vi "XNode Template Single.vi"(0 "failure in":T1 {"code" format="%.0x"}, 1 "Tag":string, 5 "Data Type":variant) -> (4 "failure out":T1 {"code" format="%.0x"}, 6 "Value":dbl, 8 "failed":bool)   [LabVIEW 2013, in "Read Exception Property.xnode"]
doc: "This VI is used to read data stored in a Variant Repository, similar to a look up table. This VI is will get an attribute of the <b>Variant Repository In</b>, with the tag name of <b>Tag</b>, and return its value on <b>Value</b>, and then return the same varient data on <b>Varient Repository Out</b>. This VI will put an error on the <b>error out</b> if the tag is not found, there is no tag when needed, or the tag was found, but of the wrong data type.\n\nRight click and Select Type for simple data types, or choose Automatic and wire in the <b>Data Type</b> to be read. If Automatic is selected, and nothing is wired to the Data Type, the type can come from the sink of the wire wired to the Value terminal.\n\nIf the a Data Type terminal is not wired, then the <b>Tag</b> must also be provided. If the data type is selected using the <b>Data Type</b> input then the tag is optional, and if empty the label associated with the data passed in will be used as the tag.\n\nReading multiple tags can be done by right clicking and choosing Read Multiple Tags.\n\n-------------\nBrian Hoover (Hooovahh)\n\nProduct Name: Variant Repository\nPackage File Name: lava_lib_variant_repository\nPackage Version: 1.0.1.11\nMinimum LabVIEW Version: 11.0"
uses:
  Read Exception Property.xnode
  failure.ctl
  <vilib>/Utility/VariantDataType/VariantType.lvlib
  failure.lvlib
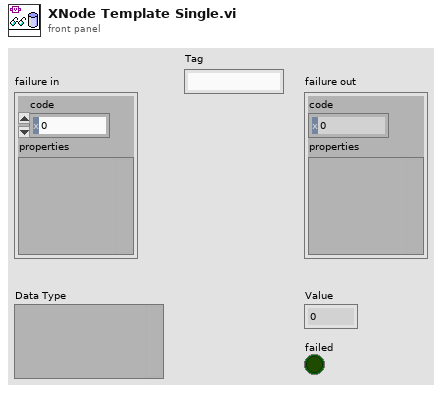
[diagram p1: front panel]
types:
  T1 = typedef "failure.lvlib/failure.ctl" = cluster{"code":i32, "properties":variant}
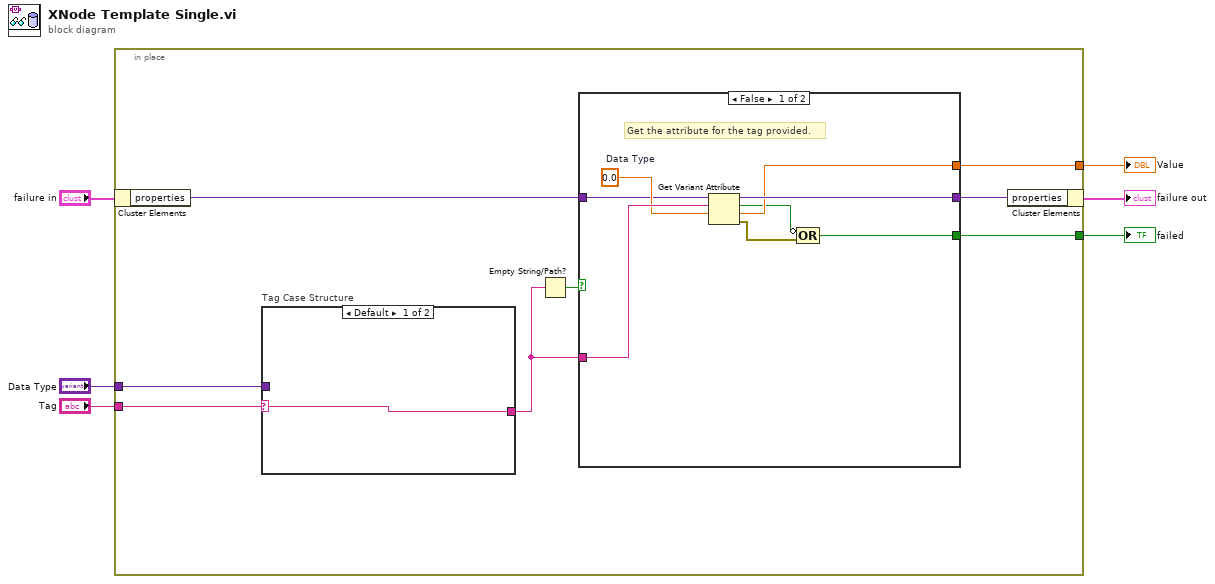
[diagram p0: block diagram]
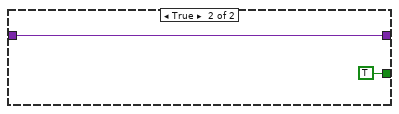
[diagram p2: hidden frame]
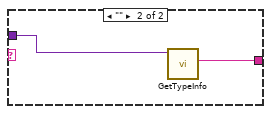
[diagram p3: hidden frame]
diagram:
  n1 = in-place {
    in-place-border: "Tag" -> [w14]
    in-place-border: [w13] -> w5
    in-place-border: "Data Type" -> [w12]
    in-place-border: [w7] -> w1
    n2 = in-place-cluster #1("failure in") -> ("properties"=w11:variant)
    n3 = case "Tag Case Structure" shown="Default" w14 {
      selector: w14 -> [w25 _]
      tunnel: w12 -> [_ w27]
      tunnel: [w25 w26] -> w9
      frame Default {
      }
      frame "" {
        n4 = call <vilib>:"GetTypeInfo.vi"("Variant"=w27) -> ("Name"=w26:string)  [unwired: 6 in, 4 out]
      }
    }
    n5 = Empty String/Path?(string/path=w9) -> (empty?=w8:bool)
    n6 = case shown="False" w8 {
      tunnel: w11 -> [w18 w24]
      tunnel: [w22 w24] -> w10
      tunnel: [w21 _] -> w13
      tunnel: w9 -> [w20 _]
      tunnel: [w15 TRUE] -> w7
      frame False {
        w19 = 0.0  # Data Type
        # "Get the attribute for the tag provided."
        n7 = Get Variant Attribute ("Read Variant Attribute")(Variant=w18, name=w20, default value (empty Variant)=w19) -> (duplicate Variant=w22:variant, found=w17:bool, value=w21:dbl, error out=w16:errorcluster)  [unwired: 1 in]
        n8 = Compound Arithmetic op=OR(invert w17, w16) -> (w15:bool)
      }
      frame True {
      }
    }
    n9 = in-place-cluster #1("properties"=w10) -> (→"failure out":T1)
  }
  "Value" <- w5
  "failed" <- w1
